vi "Check All Instances Done.vi"(8 "error in (no error)":errorcluster, 11 "Waveform Log in":refnum<class "Waveform Log.lvclass">) -> (0 "error out":errorcluster, 3 "Waveform Log out":refnum<class "Waveform Log.lvclass">)   [LabVIEW 2015, in "Waveform Log.lvclass"]
uses:
  Waveform Log.lvclass
  Waveform Log.lvclass/Waveform Log.ctl
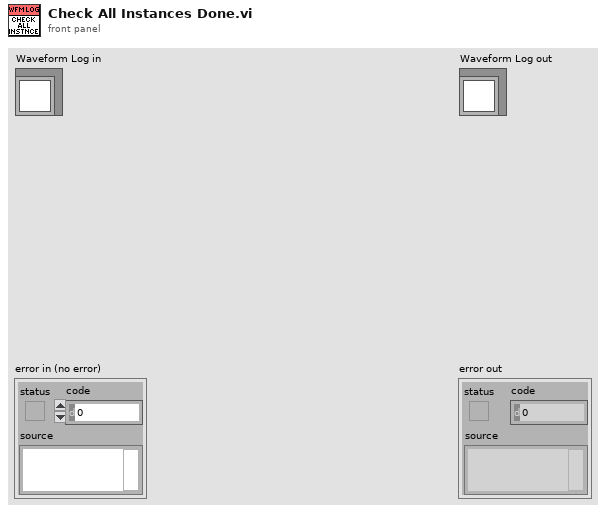
[diagram p1: front panel]
types:
  T1 = typedef "Waveform Log.lvclass/Log Instance.ctl" = cluster{"Segmented Log":refnum<data-value>, "Log Waveforms":T2[], "Log Start":timestamp, "Log Stop":timestamp, "Start Trigger Time":timestamp, "Stop Trigger Time":timestamp, "Time of Last Write":timestamp, "Timeout":dbl, "Stop cmd received":bool}
  T2 = typedef "Waveform Log.lvclass/Log Instance Waveform.ctl" = cluster{"Wfm Info":T3, "Count / Instance":i32, "Previous Segment":u64, "Wfm Complete?":bool, "Last Sample Logged":timestamp, "Data Logged":bool, "Log segmented":bool}
  T3 = typedef "Waveform Log.lvclass/Waveform Information.ctl" = cluster{"Name":string, "Wfm Data Type":T4, "Decimation":u32}
  T4 = typedef "Waveform Log.lvclass/Waveform Data Type.ctl" = enum16{"Double", "ComplexDouble"}
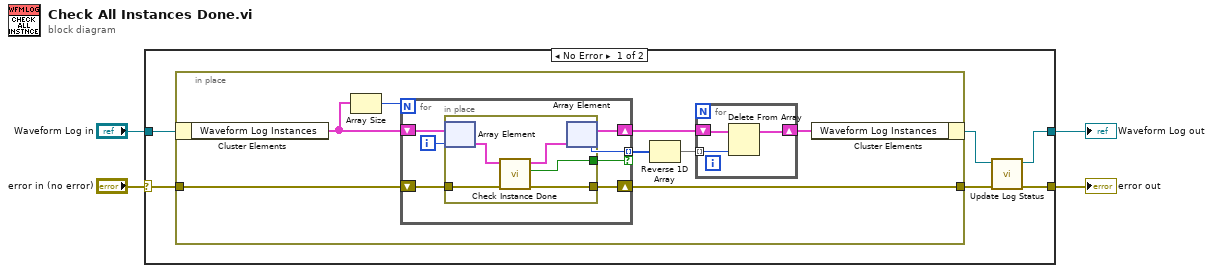
[diagram p0: block diagram]
diagram:
  n1 = case shown="No Error" "error in (no error)" {
    selector: "error in (no error)" -> [w10 w35]
    tunnel: [w5 w35] -> w3
    tunnel: [w6 w34] -> w1
    tunnel: "Waveform Log in" -> [w9 w34]
    frame No Error {
      n2 = in-place {
        in-place-border: w10 -> [w17]
        in-place-border: [w11] -> w7
        n3 = in-place-cluster #1(w9) -> ("Waveform Log Instances"=w15:T1[])
        n4 = Array Size(array=w15) -> (size(s)=w18:i32)
        n5 = for {
          N: w18 -> [_]
          shift-right: [w24] -> w14
          shift-left: w15 -> [w28]
          shift-right: [w25] -> w11
          shift-left: w17 -> [w26]
          tunnel: [w22] -> w16 mode=indexing if=w23
          i -> [w27]
          n6 = in-place {
            in-place-border: w26 -> [w32]
            in-place-border: [w31] -> w25
            in-place-border: [w29] -> w23
            n7 = in-place-array #2(w28, w27) -> (w33:T1)
            n8 = call "Check Instance Done.vi"("error in (no error)"=w32, "Log Instance in"=w33) -> ("error out"=w31:errorcluster, "Done?"=w29:bool, "Log Instance out"=w30:T1)  [unwired: 7 in]
            n9 = in-place-array #2(w30) -> (w24:T1[], w22:i32)
          }
        }
        n10 = Reverse 1D Array(array=w16) -> (reversed array=w13:i32[])
        n11 = for {
          shift-right: [w20] -> w12
          shift-left: w14 -> [w21]
          tunnel: w13 -> [w19] mode=indexing
          n12 = Delete From Array(array=w21, index=w19) -> (array with subset deleted=w20:T1[])  [unwired: 1 in, 1 out]
        }
        n13 = in-place-cluster #1("Waveform Log Instances"=w12) -> (w8:refnum<class "Waveform Log.lvclass">)
      }
      n14 = call "Update Log Status.vi"("error in (no error)"=w7, "Waveform Log in"=w8) -> ("error out"=w5:errorcluster, "Waveform Log out"=w6:refnum<class "Waveform Log.lvclass">)  [unwired: 8 in]
    }
    frame Error {
    }
  }
  "error out" <- w3
  "Waveform Log out" <- w1
